vi "GUIDs For Refresh.vi"(9 "error in (no error)":errorcluster) -> (1 "error out":errorcluster, 3 "Initialize":T1={"Paths"=["path 1", "path 2", "path 3", "path 4", "path 5"], "Rectangles"=["rect 1", "rect 2", "rect 3", "rect 4", "rect 5"], "Funnels"=["funnel 1", "funnel 2", "funnel 3", "funnel 4", "funnel 5"], "Dots"=[]})   [LabVIEW 2019]
uses:
  Setting Database/Typedefs/PrivateEvents--Setting Database.Refresh.ctl
  Setting Database/Setting Database.lvclass
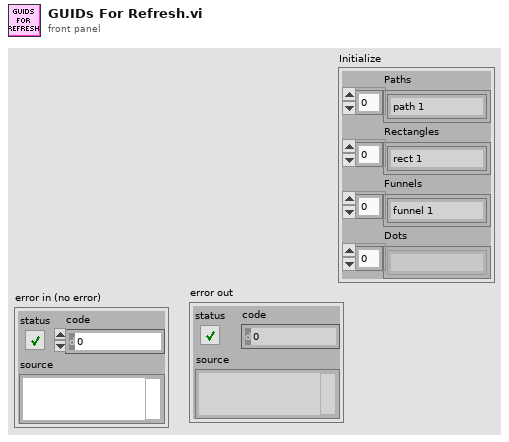
[diagram p1: front panel]
types:
  T1 = typedef "Setting Database.lvclass/PrivateEvents--Setting Database.Refresh.ctl" = cluster{"Paths":string[], "Rectangles":string[], "Funnels":string[], "Dots":string[]}
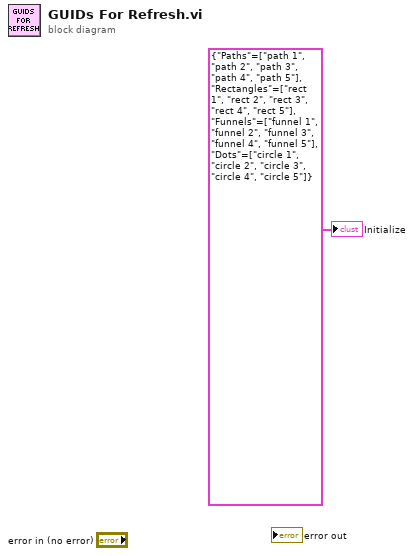
[diagram p0: block diagram]
diagram:
  "Initialize" <- T1 {"Paths"=["path 1", "path 2", "path 3", "path 4", "path 5"], "Rectangles"=["rect 1", "rect 2", "rect 3", "rect 4", "rect 5"], "Funnels"=["funnel 1", "funnel 2", "funnel 3", "funnel 4", "funnel 5"], "Dots"=["circle 1", "circle 2", "circle 3", "circle 4", "circle 5"]} ("Initialize")
